vi "Auto Set LEDs.vi"(10 "LED State":bool, 11 "Run?":bool) -> (3 "Done":bool)   [LabVIEW 2013]
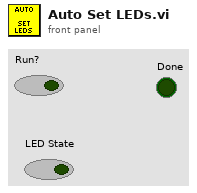
[diagram p1: front panel]
types:
  T1 = typedef "WPI_DigitalOutputDevRef.ctl" = cluster{"Digital Module":T2, "DIO Channel":T3, "DevStatus":errorcluster}
  T2 = typedef "FPGA_TypedefDigitalModule.ctl" = enum16{"Digital Module 1", "Digital Module 2"}
  T3 = typedef "FPGA_DIOChannel.ctl" = enum8{"DIO 1", "DIO 2", "DIO 3", "DIO 4", "DIO 5", "DIO 6", "DIO 7", "DIO 8", "DIO 9", "DIO 10", "DIO 11", "DIO 12", "DIO 13", "DIO 14", "Invalid"}
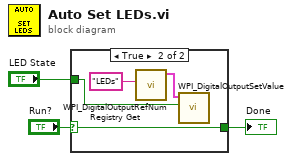
[diagram p0: block diagram]
diagram:
  n1 = case shown="True" "Run?" {
    selector: "Run?" -> [w4 w5]
    tunnel: [w4 w5] -> w2
    tunnel: "LED State" -> [_ w6]
    frame False {
    }
    frame True {
      n2 = call <vilib>:"WPI_DigitalOutputRefNum Registry Get.vi"("refnum name"="LEDs") -> ("DigitalOutputDevRef"=w8:T1)  [unwired: 9 in, 1 out]
      n3 = call <vilib>:"WPI_DigitalOutputSetValue.vi"("Value"=w6, "DigitalOutputDevRef"=w8) -> ()  [unwired: 8 in, 2 out]
    }
  }
  "Done" <- w2
